vi "Create piece.vi"(10 "Piece color":T1, 11 "Piece type":T2) -> (3 "Piece out":refnum<class "Piece.lvclass">)   [LabVIEW 2016, in "Chesslib.lvlib" / "Piece.lvclass"]
uses:
  Piece.lvclass
  typedef/Piece type.ctl
  typedef/Color.ctl
  Pawn/Pawn.lvclass
  C:/Users/GRTaggJ/Documents/Projects/chesslib/Pieces/Piece/Piece.lvclass
  Bishop/Bishop.lvclass
  Knight/Knight.lvclass
  Rook/Rook.lvclass
  Queen/Queen.lvclass
  King/King.lvclass
  Piece.lvclass/Piece.ctl
  Chesslib.lvlib
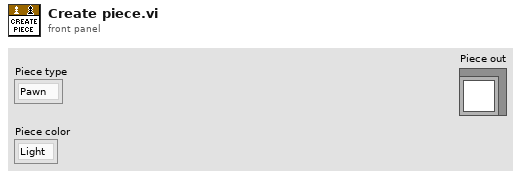
[diagram p1: front panel]
types:
  T1 = typedef "Chesslib.lvlib/Color.ctl" = enum16{"Light", "Dark"}
  T2 = typedef "Chesslib.lvlib/Piece type.ctl" = enum16{"Pawn", "Bishop", "Knight", "Rook", "Queen", "King"}
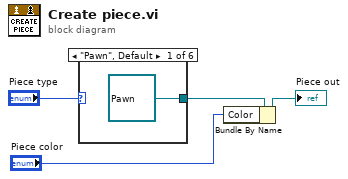
[diagram p0: block diagram]
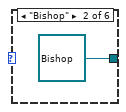
[diagram p2: hidden frame]
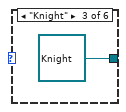
[diagram p3: hidden frame]
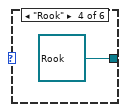
[diagram p4: hidden frame]
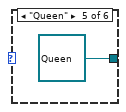
[diagram p5: hidden frame]
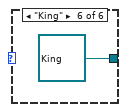
[diagram p6: hidden frame]
diagram:
  n1 = case shown="\"Pawn\", Default" "Piece type" {
    tunnel: [refnum<class "Pawn.lvclass"> refnum ("Chesslib.lvlib:Pawn.lvclass") refnum<class "Bishop.lvclass"> refnum ("Chesslib.lvlib:Bishop.lvclass") refnum<class "Knight.lvclass"> refnum ("Chesslib.lvlib:Knight.lvclass") refnum<class "Rook.lvclass"> refnum ("Chesslib.lvlib:Rook.lvclass") refnum<class "Queen.lvclass"> refnum ("Chesslib.lvlib:Queen.lvclass") refnum<class "King.lvclass"> refnum ("Chesslib.lvlib:King.lvclass")] -> w3
    frame "Pawn", Default {
    }
    frame "Bishop" {
    }
    frame "Knight" {
    }
    frame "Rook" {
    }
    frame "Queen" {
    }
    frame "King" {
    }
  }
  n2 = Bundle By Name(cluster=w3, "Color"="Piece color") -> (→"Piece out":refnum<class "Piece.lvclass">)
